vi "Set PID.vi"(5 "Output #":i32=1, 6 "D":dbl, 7 "P manual":dbl, 8 "error in (no error)":errorcluster, 9 "I":dbl, 10 "P":dbl, 11 "Cryo-Con Driver in":refnum<class "Cryo-Con Driver.lvclass">) -> (0 "error out":errorcluster, 3 "Cryo-Con Driver out":refnum<class "Cryo-Con Driver.lvclass">)   [LabVIEW 2021, in "Cryo-Con Driver.lvclass"]
uses:
  Cryo-Con Driver.lvclass
  C:/GitHub/NHMFL_Core/Libraries/Instruments/VISA Instrument/VISA Instrument.lvclass
  C:/GitHub/NHMFL_Core/Libraries/Instruments/Temperature Controller Driver/Temperature Controller Driver.lvclass
  VISA Instrument/VISA Instrument.lvclass/VISA Instrument.ctl
  VISA Instrument/Read VISA resource.vi
  VISA Instrument/Write VISA resource.vi
  Temperature Controller Driver/Read T controller configuration.vi
  Cryo-Con Driver.lvclass/Cryo-Con Driver.ctl
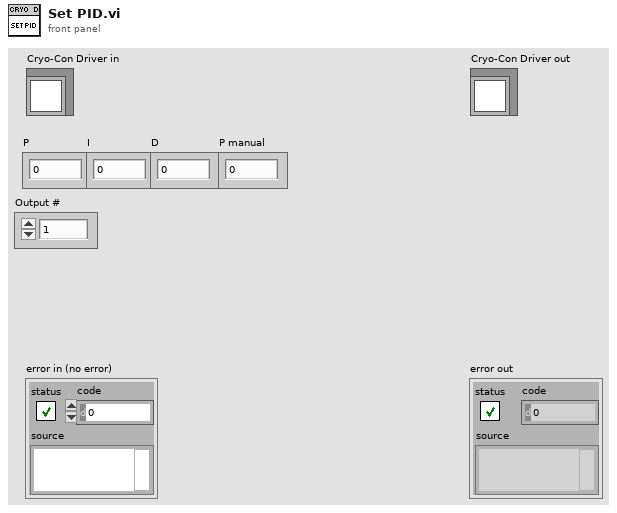
[diagram p1: front panel]
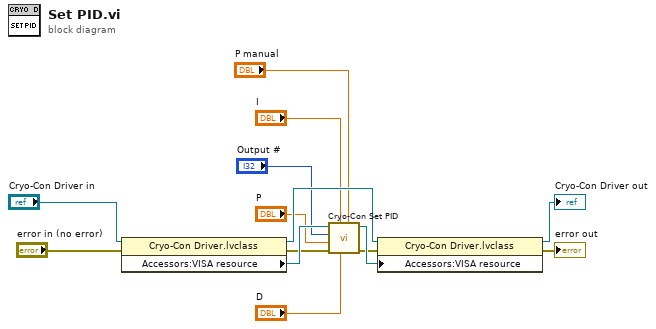
[diagram p0: block diagram]
diagram:
  n1 = property class="Cryo-Con Driver.lvclass"(reference="Cryo-Con Driver in", error in="error in (no error)") -> (reference out=w9:refnum<class "Cryo-Con Driver.lvclass">, error out=w8:errorcluster, "Accessors:VISA resource"=w12:refnum<visa-resource-name>)
  n2 = call "Cryo-Con Set PID.vi"("P manual"="P manual", "D"="D", "I"="I", "Error In"=w8, "P"="P", "Loop number"="Output #", "VISA resource name"=w12) -> ("Error Out"=w7:errorcluster, "VISA resource name out"=w11:refnum<visa-resource-name>)  [unwired: 3 in]
  n3 = property class="Cryo-Con Driver.lvclass"(reference=w9, error in=w7, "Accessors:VISA resource"=w11) -> (reference out=→"Cryo-Con Driver out":refnum<class "Cryo-Con Driver.lvclass">, error out=→"error out":errorcluster)
